vi "Run Bfr Rx - Handle Offset.vi"(7 "Offset in":u64, 8 "error in (no error)":errorcluster, 10 "Data":u8[](array[numeric]), 11 "Data Buffer in":u64 format="%016x") -> (0 "error out":errorcluster, 2 "Data Size":u64, 3 "Data Buffer out":u64 format="%016x", 5 "Offset out":u64)   [LabVIEW 2019, in "UDP-Custom-Device Engine.lvlib"]
uses:
  UDP-Custom-Device Engine.lvlib
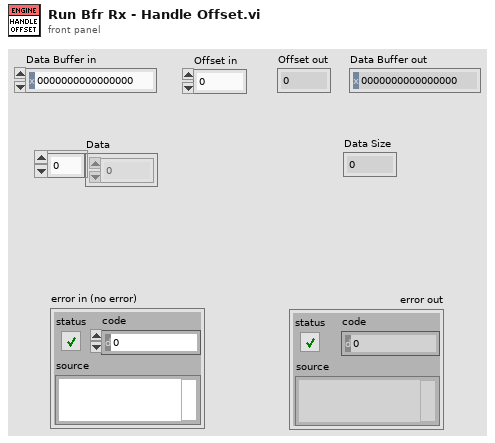
[diagram p1: front panel]
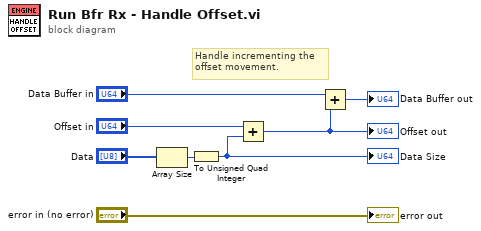
[diagram p0: block diagram]
diagram:
  # "Handle incrementing the\noffset movement."
  n1 = Array Size(array="Data") -> (size(s)=w2:i32)
  n2 = To Unsigned Quad Integer(1:w2) -> (0:w1:u64)
  "Data Size" <- w1
  n3 = Add(x="Offset in", y=w1) -> (x+y=w3:u64)
  "Offset out" <- w3
  n4 = Add(x="Data Buffer in", y=w3) -> (x+y=→"Data Buffer out":u64)
  "error out" <- "error in (no error)"
